vi "行上色模块.vi"(8 "error in (no error)":errorcluster caption="错误输入（无错误）", 9 "点":T2 caption="表格点", 10 "初始化":T1={"颜色"={"选中颜色"=2764799, "未选中颜色"=16777216}, "表格引用"=refnum, "列数"=0, "上次的行"=0}, 11 "枚举":enum16{"初始化", "上色", "释放", "无"}(ring)) -> (0 "error out":errorcluster caption="错误输出", 3 "信息输出":T1)   [LabVIEW 2014, in "表格.lvlib" / "表格上色.lvlib"]
uses:
  <vilib>/Utility/miscctls.llb/LVPositionTypeDef.ctl
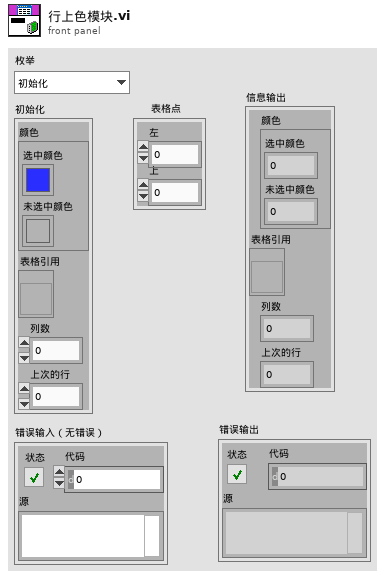
[diagram p1: front panel]
types:
  T1 = cluster{"颜色":cluster{"选中颜色":u32, "未选中颜色":u32}, "表格引用":refnum<vi>, "列数":i32, "上次的行":i32}
  T2 = typedef "LVPositionTypeDef.ctl" = cluster{"Left":i32, "Top":i32}
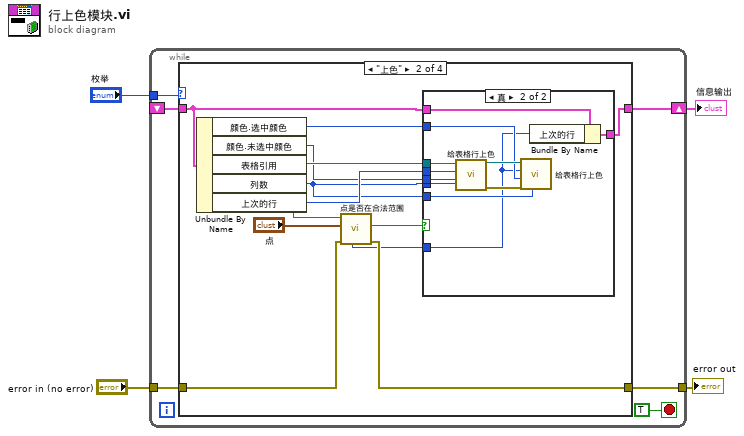
[diagram p0: block diagram]
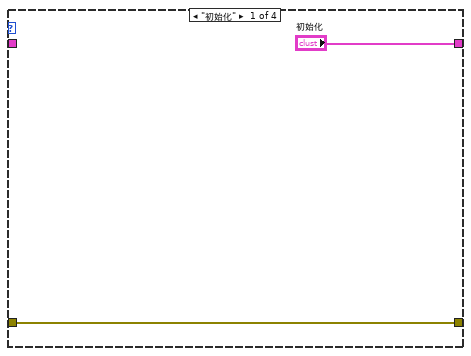
[diagram p2: hidden frame]
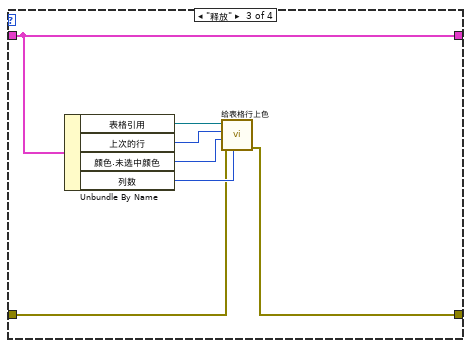
[diagram p4: hidden frame]
diagram:
  n1 = while {
    shift-right: [w10] -> w1
    shift-left: _ -> [w9]
    tunnel: "error in (no error)" -> [w8]
    tunnel: [w7] -> w3
    tunnel: "枚举" -> [w6]
    stop <- TRUE stop-if-true
    n2 = case shown="\"上色\"" w6 {
      tunnel: ["初始化" w13 w37 w44] -> w10
      tunnel: w9 -> [_ w14 w37 w44]
      tunnel: w8 -> [w11 w23 w39 w45]
      tunnel: [w11 w22 w38 w45] -> w7
      frame "初始化" {
      }
      frame "上色" {
        n3 = Unbundle By Name(w14) -> ("颜色.选中颜色"=w18:u32, "颜色.未选中颜色"=w19:u32, "表格引用"=w21:refnum<vi>, "列数"=w15:i32, "上次的行"=w20:i32)
        n4 = call "点是否在合法范围.vi"("错误输入（无错误）"=w23, "点"="点", "Table输入"=w21) -> ("错误输出"=w22:errorcluster, "是否在范围"=w16:bool, "行"=w17:i32)  [unwired: 4 in, 2 out]
        n5 = case shown="真" w16 {
          tunnel: w21 -> [_ w36]
          tunnel: w20 -> [_ w35]
          tunnel: w15 -> [_ w34]
          tunnel: w19 -> [_ w33]
          tunnel: w18 -> [_ w30]
          tunnel: w17 -> [_ w26]
          tunnel: w15 -> [_ w29]
          tunnel: w14 -> [w25 w28]
          tunnel: [w25 w27] -> w13
          frame False {
          }
          frame True {
            n6 = call "给表格行上色.vi"("列数"=w34, "颜色"=w33, "行输入"=w35, "引用输入"=w36) -> ("错误输出"=w32:errorcluster, "引用输出"=w31:refnum<vi>)  [unwired: 5 in, 1 out]
            n7 = call "给表格行上色.vi"("列数"=w29, "错误输入（无错误）"=w32, "颜色"=w30, "行输入"=w26, "引用输入"=w31) -> ()  [unwired: 4 in, 3 out]
            n8 = Bundle By Name(cluster=w28, "上次的行"=w26) -> (w27:T1)
          }
        }
      }
      frame "释放" {
        n9 = Unbundle By Name(w37) -> ("表格引用"=w43:refnum<vi>, "上次的行"=w40:i32, "颜色.未选中颜色"=w41:u32, "列数"=w42:i32)
        n10 = call "给表格行上色.vi"("列数"=w42, "错误输入（无错误）"=w39, "颜色"=w41, "行输入"=w40, "引用输入"=w43) -> ("错误输出"=w38:errorcluster)  [unwired: 4 in, 2 out]
      }
      frame "无", Default {
      }
    }
  }
  "error out" <- w3
  "信息输出" <- w1
